vi "read_mod.vi"(8 "error in (no error)":errorcluster, 11 "msg":T7) -> (0 "error out":errorcluster, 1 "LINX Resource":T1, 2 "Data":u8[](array[numeric]), 3 "string":string)   [LabVIEW 2021]
uses:
  CTLs/msg.ctl
  <vilib>/MakerHub/LINX/Private/Type Defs/LINX Ref.ctl
  <vilib>/MakerHub/LINX/Private/Type Defs/Platform.ctl
  <vilib>/MakerHub/LINX/Private/Type Defs/Interface.ctl
  <vilib>/MakerHub/LINX/Private/Device/Type Defs/LINX Device Config.ctl
  <vilib>/MakerHub/LINX/Private/Device/Type Defs/TCP Config.ctl
  <vilib>/MakerHub/LINX/Private/Device/Type Defs/Channels.ctl
  Global 1.vi
  <vilib>/MakerHub/LINX/LMH-LINX.lvlib
  <vilib>/MakerHub/LINX/Private/Device/Device.lvlib
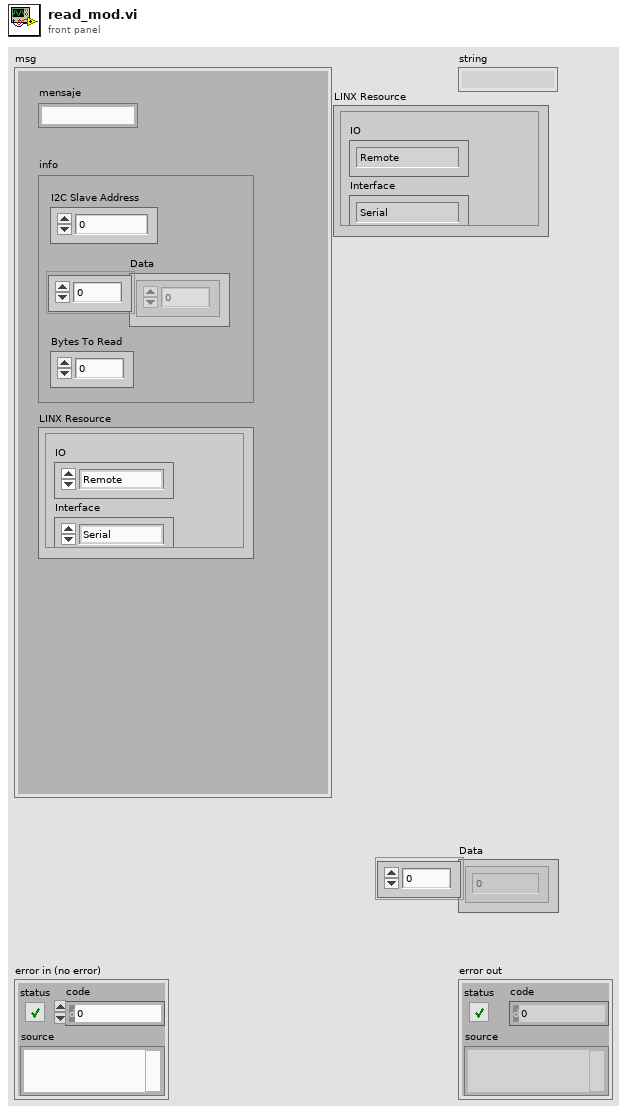
[diagram p1: front panel]
types:
  T1 = typedef "LMH-LINX.lvlib/LINX Ref.ctl" = cluster{"IO":T2, "Interface":T3, "LINX Device Config":T4}
  T2 = typedef "LMH-LINX.lvlib/Platform.ctl" = enum16{"Remote", "Local"}
  T3 = typedef "LMH-LINX.lvlib/Interface.ctl" = enum16{"Serial", "TCP"}
  T4 = typedef "LMH-LINX.lvlib/Device.lvlib/LINX Device Config.ctl" = cluster{"Interface":T3, "COM Port":refnum<visa-resource-name>, "TCP Configuration":T5, "Device Family":u8, "Device ID":u8, "Device Name":string, "TCP Ref":refnum<k5>, "Channels":T6}
  T5 = typedef "LMH-LINX.lvlib/Device.lvlib/TCP Config.ctl" = cluster{"IP Address":string, "Port":u16}
  T6 = typedef "LMH-LINX.lvlib/Channels.ctl" = cluster{"DI":u8[], "DO":u8[], "AI":u8[], "AO":u8[], "PWM":u8[], "QE":u8[], "UART":u8[], "I2C 2":u8[], "SPI":u8[], "CAN":u8[], "Servo":u8[], "AI Ref (V)":dbl, "AI Resolution (Bits)":u8, "AO Ref (V)":dbl, "AO Resolution (Bits)":u8}
  T7 = typedef "msg.ctl" = cluster{"mensaje":string, "info":cluster{"I2C Slave Address ":u8, "Data":u8[], "Bytes To Read":u8}, "LINX Resource":T1}
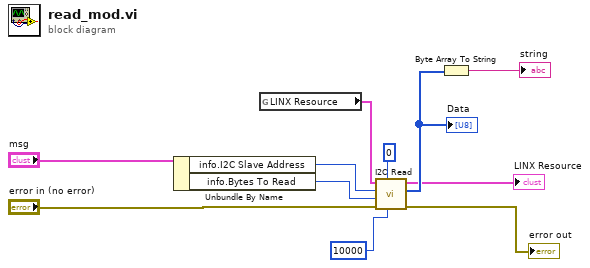
[diagram p0: block diagram]
diagram:
  n1 = Unbundle By Name("msg") -> ("info.I2C Slave Address"=w6:u8, "info.Bytes To Read"=w7:u8)
  n2 = global read "Global 1.vi" "LINX Resource"() -> (w3:T1)
  n3 = call <vilib>:"I2C Read.vi"("Timeout (1000 ms)"=u16 10000, "I2C Channel"=u8 0, "Error In"="error in (no error)", "Bytes To Read"=w7, "I2C Slave Address (0)"=w6, "LINX Resource"=w3) -> ("Error Out"=→"error out":errorcluster, "Data"=w8:u8[], "LINX Resource"=→"LINX Resource":T1)  [unwired: 3 in]
  "Data" <- w8
  n4 = Byte Array To String(unsigned byte array=w8) -> (string=→"string":string)
